vi "Replace State.vi"(0 "Tosca in":refnum<class "Parameters.lvclass">, 5 "stateIndex":i32, 7 "State":refnum<class "State.lvclass">) -> (4 "Tosca out":refnum<class "Parameters.lvclass">)   [LabVIEW 2020, in "Parameters.lvclass"]
uses:
  Parameters.lvclass
  State/State.lvclass
  Parameters.lvclass/Parameters.ctl
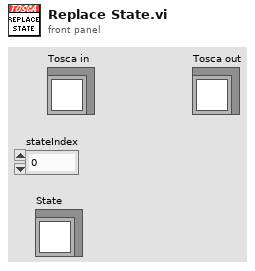
[diagram p1: front panel]
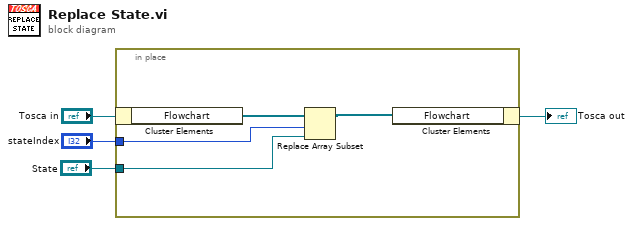
[diagram p0: block diagram]
diagram:
  n1 = in-place {
    in-place-border: "stateIndex" -> [w6]
    in-place-border: "State" -> [w5]
    n2 = in-place-cluster #1("Tosca in") -> ("Flowchart"=w8:refnum<class "State.lvclass">[])
    n3 = Replace Array Subset(array=w8, new element=w5, index=w6) -> (w7:refnum<class "State.lvclass">[])
    n4 = in-place-cluster #1("Flowchart"=w7) -> (→"Tosca out":refnum<class "Parameters.lvclass">)
  }
